vi "Set.vi"() -> ()   [LabVIEW 2010]
uses:
  <vilib>/addons/database/Connection.llb/DB Tools Open Connec (String).vi
  <vilib>/addons/database/Connection.llb/Conn Execute.vi
  <vilib>/addons/database/Recordset.llb/Rec Destroy - Connection.vi
  <vilib>/addons/database/NI_Database_API.lvlib
panel:
  out "exec_time":timestamp
  out "error in (no error)":errorcluster
  out "Database":string
  out "error in (no error) 2":errorcluster
  out "submit_time":timestamp
  out "exp_id":i32
  out "XML-String-out":string
  out "Status":string
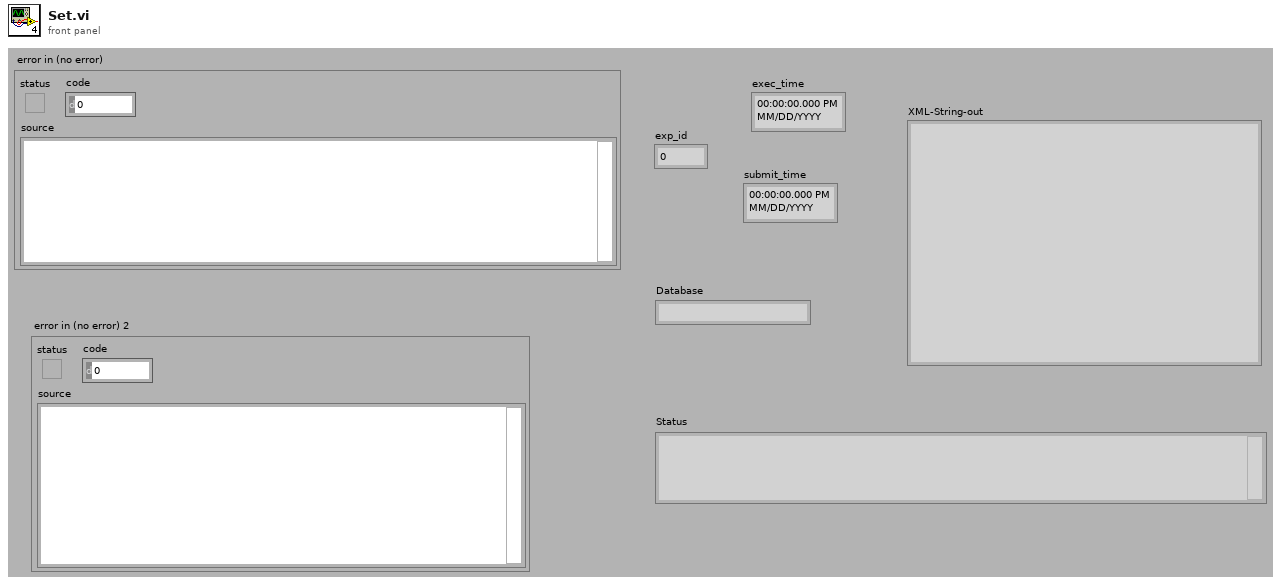
[diagram p1: front panel]
types:
  T1 = typedef "NI_Database_API.lvlib/Conn ObjectReference.ctl" = refnum<k1>
  T2 = typedef "NI_Database_API.lvlib/Rec ObjectReference.ctl" = refnum<k1>
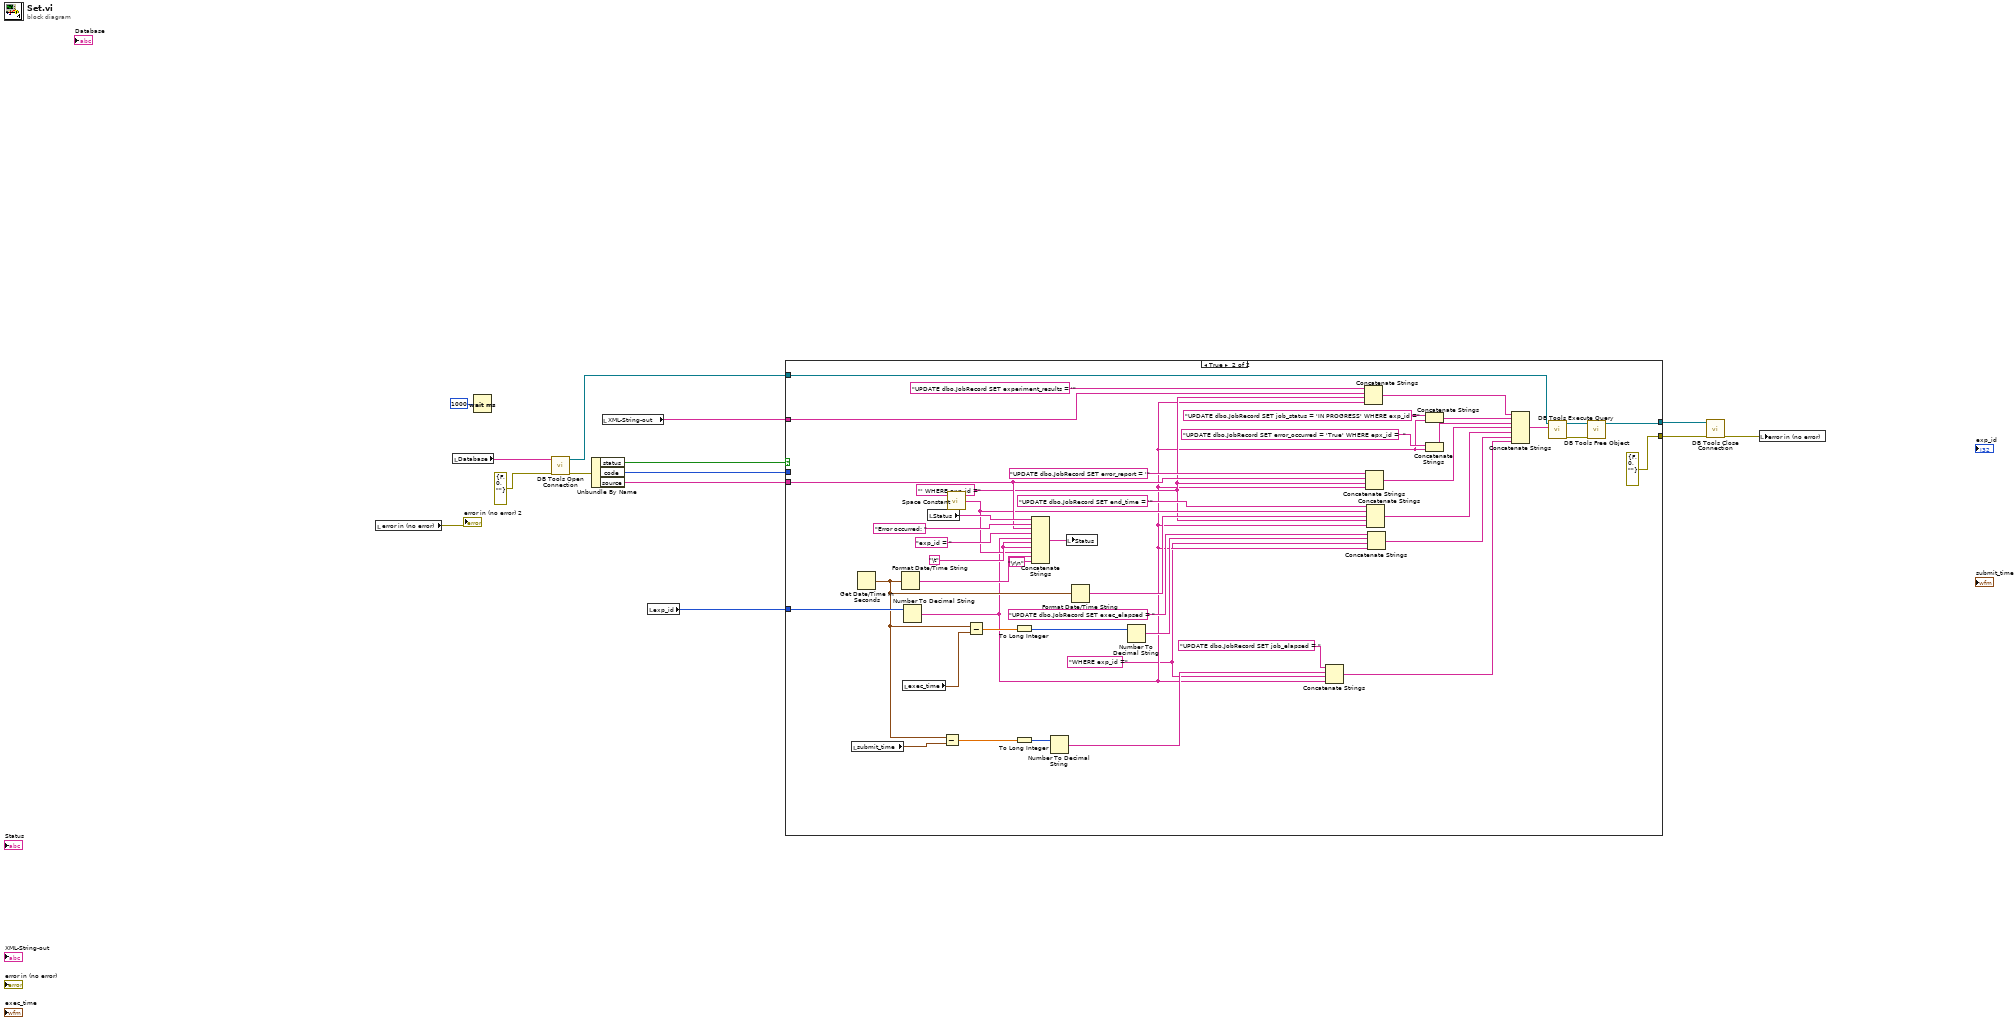
[diagram p0: block diagram]
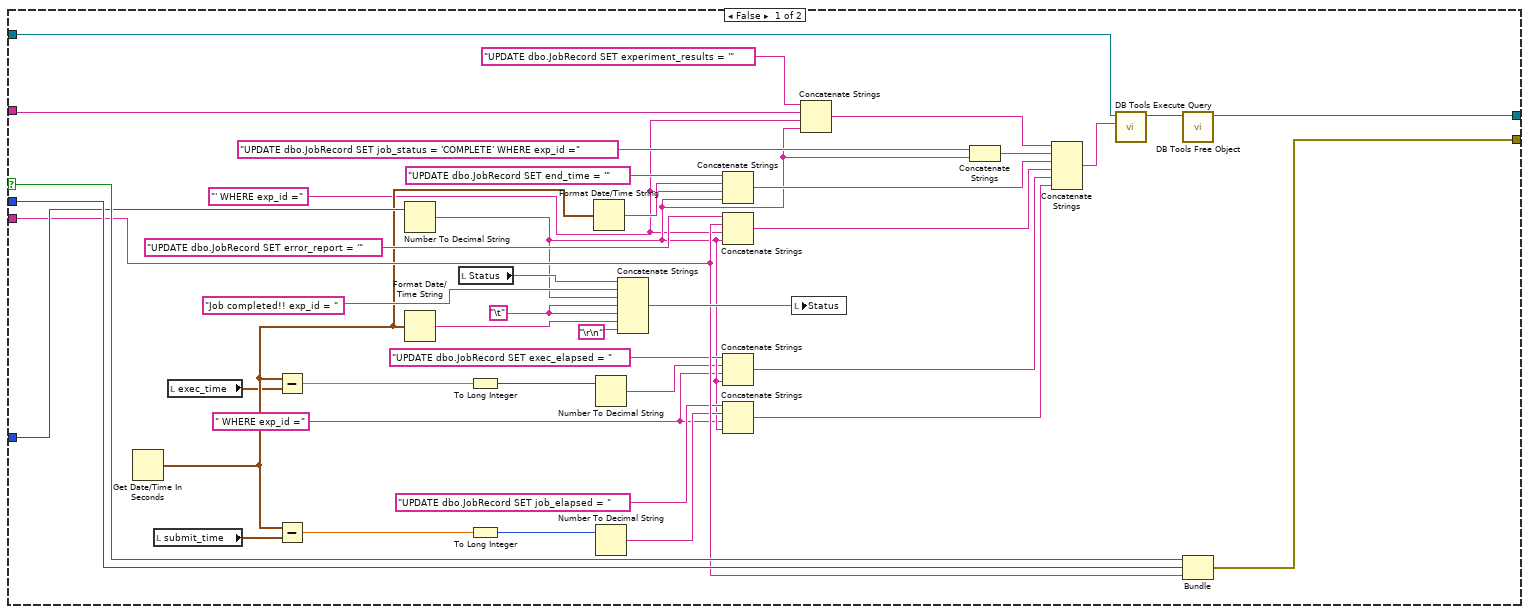
[diagram p2: hidden frame]
diagram:
  n1 = local read "error in (no error)"() -> (→"error in (no error) 2":errorcluster)
  n2 = local read "Database"() -> (w14:string)
  n3 = Wait (ms)(milliseconds to wait=u32 1000) -> ()  [unwired: 1 out]
  n4 = call-poly <vilib>:"DB Tools Open Connection.vi"("error in (no error)"=errorcluster {"status"=FALSE, "code"=0, "source"=""}, "connection information"=w14) -> ("error out"=w3:errorcluster, "connection reference"=w7:T1)  [unwired: 6 in]
  n5 = Unbundle By Name(w3) -> ("status"=w12:bool, "code"=w6:i32, "source"=w10:string)
  n6 = local read "XML-String-out"() -> (w9:string)
  n7 = local read "exp_id"() -> (w8:i32)
  n8 = case shown="True" w12 {
    selector: w12 -> [w55 _]
    tunnel: w6 -> [w54 _]
    tunnel: w10 -> [w32 w78]
    tunnel: [w53 errorcluster {"status"=FALSE, "code"=0, "source"=""} ("error in (no error)")] -> w4
    tunnel: w7 -> [w52 w91]
    tunnel: [w50 w82] -> w5
    tunnel: w9 -> [w42 w90]
    tunnel: w8 -> [w41 w89]
    frame False {
      w16 = "' WHERE exp_id =" ("string")
      w34 = "\t"
      w17 = " WHERE exp_id ="
      n9 = Get Date/Time In Seconds() -> (seconds since 1Jan1904=w24:timestamp)
      n10 = local read "submit_time"() -> (w21:timestamp)
      n11 = local read "exec_time"() -> (w22:timestamp)
      n12 = Subtract(x=w24, y=w22) -> (x-y=w30:dbl)
      n13 = Subtract(x=w24, y=w21) -> (x-y=w29:dbl)
      n14 = Number To Decimal String(number=w41) -> (decimal integer string=w25:string)  [unwired: 1 in]
      n15 = Format Date/Time String(seconds (now)=w24) -> (date/time string=w35:string)  [unwired: 2 in]
      n16 = local read "Status"() -> (w39:string)
      n17 = To Long Integer(number=w30) -> (32bit integer=w19:i32)
      n18 = To Long Integer(number=w29) -> (32bit integer=w18:i32)
      n19 = Format Date/Time String(seconds (now)=w24) -> (date/time string=w45:string)  [unwired: 2 in]
      n20 = Number To Decimal String(number=w19) -> (decimal integer string=w23:string)  [unwired: 1 in]
      n21 = Number To Decimal String(number=w18) -> (decimal integer string=w27:string)  [unwired: 1 in]
      n22 = Concatenate Strings(w39, "Job completed!! exp_id = " ("string"), w25, w34, w34, w35, "\r\n") -> (w38:string)
      n23 = Concatenate Strings("UPDATE dbo.JobRecord SET end_time = '", w45, w16, w25) -> (w49:string)
      n24 = Concatenate Strings("UPDATE dbo.JobRecord SET error_report = '" ("string"), w32, w16, w25) -> (w31:string)
      n25 = Concatenate Strings("UPDATE dbo.JobRecord SET exec_elapsed = ", w23, w17, w25) -> (w20:string)
      n26 = Concatenate Strings("UPDATE dbo.JobRecord SET job_elapsed = ", w27, w17, w25) -> (w15:string)
      n27 = local write "Status"(w38) -> ()
      n28 = Concatenate Strings("UPDATE dbo.JobRecord SET experiment_results = '", w42, w16, w25) -> (w47:string)
      n29 = Concatenate Strings("UPDATE dbo.JobRecord SET job_status = 'COMPLETE' WHERE exp_id =", w25) -> (w48:string)
      n30 = Concatenate Strings(w47, w48, w49, w31, w20, w15) -> (w40:string)
      n31 = call-poly <vilib>:"DB Tools Execute Query.vi"("SQL query"=w40, "connection reference"=w52) -> ("recordset reference"=w51:T2)  [unwired: 6 in, 1 out]
      n32 = call-poly <vilib>:"DB Tools Free Object.vi"("recordset reference"=w51) -> ("connection reference"=w50:T1)  [unwired: 9 in, 1 out]
      n33 = Bundle(w55, "code"=w54, "source"=w32) -> (w53:cluster{bool, "code":i32, "source":string})  [unwired: 1 in]
    }
    frame True {
      w57 = "WHERE exp_id =" ("string")
      w76 = "\t"
      w61 = "' WHERE exp_id ="
      n34 = local read "submit_time"() -> (w65:timestamp)
      n35 = Get Date/Time In Seconds() -> (seconds since 1Jan1904=w66:timestamp)
      n36 = Format Date/Time String(seconds (now)=w66) -> (date/time string=w73:string)  [unwired: 2 in]
      n37 = local read "exec_time"() -> (w75:timestamp)
      n38 = Number To Decimal String(number=w89) -> (decimal integer string=w60:string)  [unwired: 1 in]
      n39 = local read "Status"() -> (w80:string)
      n40 = Subtract(x=w66, y=w65) -> (x-y=w64:dbl)
      n41 = call <vilib>:"Space Constant.vi"() -> ("String"=w71:string)
      n42 = Subtract(x=w66, y=w75) -> (x-y=w70:dbl)
      n43 = To Long Integer(number=w70) -> (32bit integer=w58:i32)
      n44 = To Long Integer(number=w64) -> (32bit integer=w59:i32)
      n45 = Concatenate Strings(w80, "Error occurred: " ("Status"), w78, "exp_id = " ("string"), w60, w76, w76, w71, w73, "\r\n") -> (w79:string)
      n46 = Number To Decimal String(number=w59) -> (decimal integer string=w62:string)  [unwired: 1 in]
      n47 = local write "Status"(w79) -> ()
      n48 = Format Date/Time String(seconds (now)=w66) -> (date/time string=w72:string)  [unwired: 2 in]
      n49 = Number To Decimal String(number=w58) -> (decimal integer string=w68:string)  [unwired: 1 in]
      n50 = Concatenate Strings("UPDATE dbo.JobRecord SET job_elapsed = ", w62, w57, w60) -> (w56:string)
      n51 = Concatenate Strings("UPDATE dbo.JobRecord SET experiment_results = '", w90, w61, w60) -> (w96:string)
      n52 = Concatenate Strings("UPDATE dbo.JobRecord SET error_report = '" ("string"), w78, w61, w60) -> (w84:string)
      n53 = Concatenate Strings("UPDATE dbo.JobRecord SET end_time = '", w71, w72, w61, w60) -> (w86:string)
      n54 = Concatenate Strings("UPDATE dbo.JobRecord SET exec_elapsed = ", w68, w57, w60) -> (w67:string)
      n55 = Concatenate Strings("UPDATE dbo.JobRecord SET job_status = 'IN PROGRESS' WHERE exp_id =", w60) -> (w97:string)
      n56 = Concatenate Strings("UPDATE dbo.JobRecord SET error_occurred = 'True' WHERE epx_id =  " ("string"), w60) -> (w87:string)
      n57 = Concatenate Strings(w96, w97, w87, w84, w86, w67, w56) -> (w92:string)
      n58 = call-poly <vilib>:"DB Tools Execute Query.vi"("SQL query"=w92, "connection reference"=w91) -> ("error out"=w83:errorcluster, "recordset reference"=w98:T2)  [unwired: 6 in]
      n59 = call-poly <vilib>:"DB Tools Free Object.vi"("error in (no error)"=w83, "recordset reference"=w98) -> ("connection reference"=w82:T1)  [unwired: 8 in, 1 out]
    }
  }
  n60 = call <vilib>:"DB Tools Close Connection.vi"("error in (no error)"=w4, "connection reference"=w5) -> ("error out"=w11:errorcluster)  [unwired: 5 in]
  n61 = local write "error in (no error)"(w11) -> ()
